vi "Que_Remove.vi"(6 "Time out(-1)":i32=-1 caption="Time Out(-1)_Queue Out", 8 "error in (no error)":errorcluster caption="Error In (no error)", 11 "Queue Name":string) -> (0 "error out":errorcluster caption="Error Out", 1 "timed out":bool caption="Time Out?", 2 "Data":variant, 3 "Event":string)   [LabVIEW 2016]
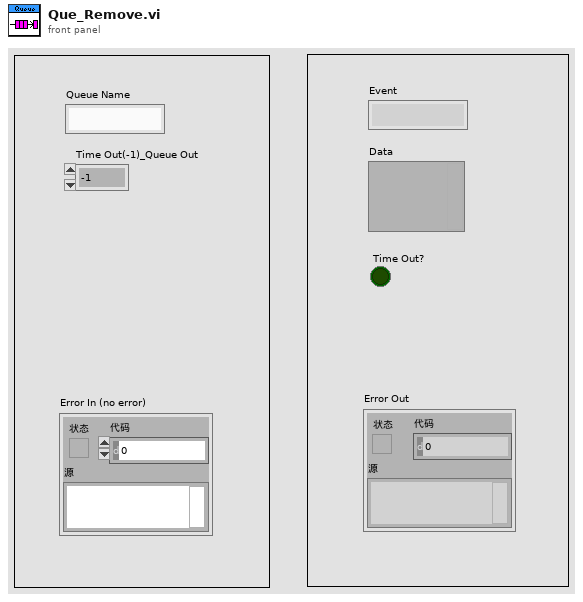
[diagram p1: front panel]
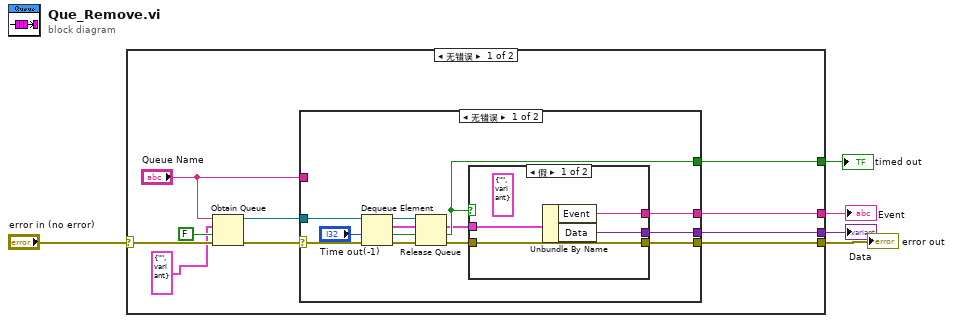
[diagram p0: block diagram]
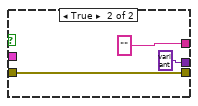
[diagram p2: hidden frame]
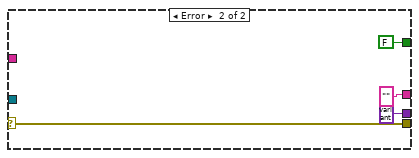
[diagram p3: hidden frame]
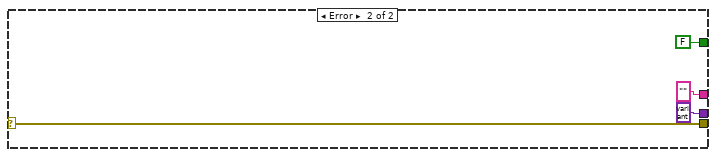
[diagram p4: hidden frame]
diagram:
  n1 = case shown="无错误" "error in (no error)" {
    selector: "error in (no error)" -> [w11 w41]
    tunnel: [w15 w41] -> w4
    tunnel: [w9 "" ("Command 2")] -> w3
    tunnel: [w8 variant ("Variant")] -> w2
    tunnel: [w7 FALSE ("timed out?")] -> w1
    frame No Error {
      n2 = Obtain Queue(name (unnamed)="Queue Name", element data type=cluster{"Event":string, "Data":variant} {"Event"="", "Data"=variant}, create if not found? (T)=FALSE ("如未找到是否创建？(T)"), error in (no error)=w11) -> (queue out=w12:refnum<queue>, error out=w10:errorcluster)  [unwired: 1 in, 1 out]
      n3 = case shown="无错误" w10 {
        selector: w10 -> [w16 w35]
        tunnel: [w26 variant ("Variant")] -> w8
        tunnel: [w25 "" ("Command 2")] -> w9
        tunnel: [w24 w35] -> w15
        tunnel: [w21 FALSE ("timed out?")] -> w7
        tunnel: "Queue Name" -> [_ _]
        tunnel: w12 -> [w23 _]
        frame No Error {
          n4 = Dequeue Element(queue=w23, timeout in ms (-1)="Time out(-1)", error in (no error)=w16) -> (queue out=w18:refnum<queue>, element=w20:cluster{"Event":string, "Data":variant}, timed out?=w21:bool, error out=w19:errorcluster)
          n5 = Release Queue(queue=w18, error in (no error)=w19) -> (error out=w17:errorcluster)  [unwired: 1 in, 2 out]
          n6 = case shown="假" w21 {
            tunnel: w20 -> [w27 _]
            tunnel: [w30 variant ("Data")] -> w26
            tunnel: [w29 "" ("Command 2")] -> w25
            tunnel: w17 -> [w28 w32]
            tunnel: [w28 w32] -> w24
            frame False {
              (unwired) cluster{"Event":string, "Data":variant} {"Event"="", "Data"=variant}
              n7 = Unbundle By Name(w27) -> ("Event"=w29:string, "Data"=w30:variant)
            }
            frame True {
            }
          }
        }
        frame Error {
        }
      }
    }
    frame Error {
    }
  }
  "error out" <- w4
  "Event" <- w3
  "Data" <- w2
  "timed out" <- w1
